vi "Write Roles.vi"(8 "error in (no error)":errorcluster, 10 "Roles":T1, 11 "5PreparePassGamePlay in":refnum<class "5PreparePassGamePlay.lvclass">) -> (0 "error out":errorcluster, 3 "5PreparePassGamePlay out":refnum<class "5PreparePassGamePlay.lvclass">)   [LabVIEW 2021, in "5PreparePassGamePlay.lvclass"]
uses:
  5PreparePassGamePlay.lvclass
  5RobotsRole_class/5RobotsRole.lvclass
  AttackerStopRole_class/AttackerStopRole.lvclass
  5PreparePassGamePlay.lvclass/5PreparePassGamePlay.ctl
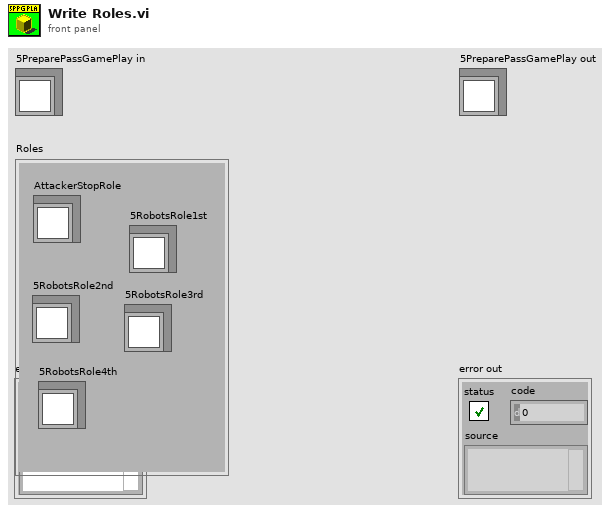
[diagram p1: front panel]
types:
  T1 = cluster{"5RobotsRole1st":refnum<class "5RobotsRole.lvclass">, "5RobotsRole2nd ":refnum<class "5RobotsRole.lvclass">, "5RobotsRole3rd":refnum<class "5RobotsRole.lvclass">, "5RobotsRole4th":refnum<class "5RobotsRole.lvclass">, "AttackerStopRole":refnum<class "AttackerStopRole.lvclass">}
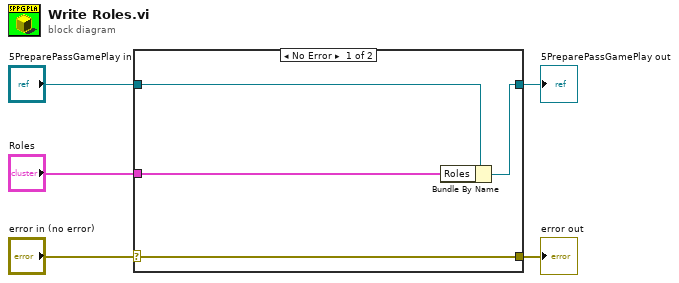
[diagram p0: block diagram]
diagram:
  n1 = case shown="No Error" "error in (no error)" {
    selector: "error in (no error)" -> [w9 w10]
    tunnel: [w9 w10] -> w4
    tunnel: [w7 w11] -> w2
    tunnel: "5PreparePassGamePlay in" -> [w8 w11]
    tunnel: "Roles" -> [w6 _]
    frame No Error {
      n2 = Bundle By Name(cluster=w8, "Roles"=w6) -> (w7:refnum<class "5PreparePassGamePlay.lvclass">)
    }
    frame Error {
    }
  }
  "error out" <- w4
  "5PreparePassGamePlay out" <- w2
